vi "Create Message Accessors.vi"(6 "Enum Parameters":T1[](array[typedef]), 7 "Message parameters":T2[](array[typedef]), 8 "error in (no error)":errorcluster, 11 "Library":refnum<vi>) -> (0 "error out":errorcluster, 3 "Library":refnum<vi>)   [LabVIEW 2019, in "gRPC Template Creation Utility.lvlib"]
uses:
  gRPC Template Creation Utility.lvlib
  TypeDefs/Message Metadata (Scripting).ctl
  TypeDefs/Message Element Metadata (Scripting).ctl
  TypeDefs/Message Element Type.ctl
  TypeDefs/Enum Metadata (Scripting).ctl
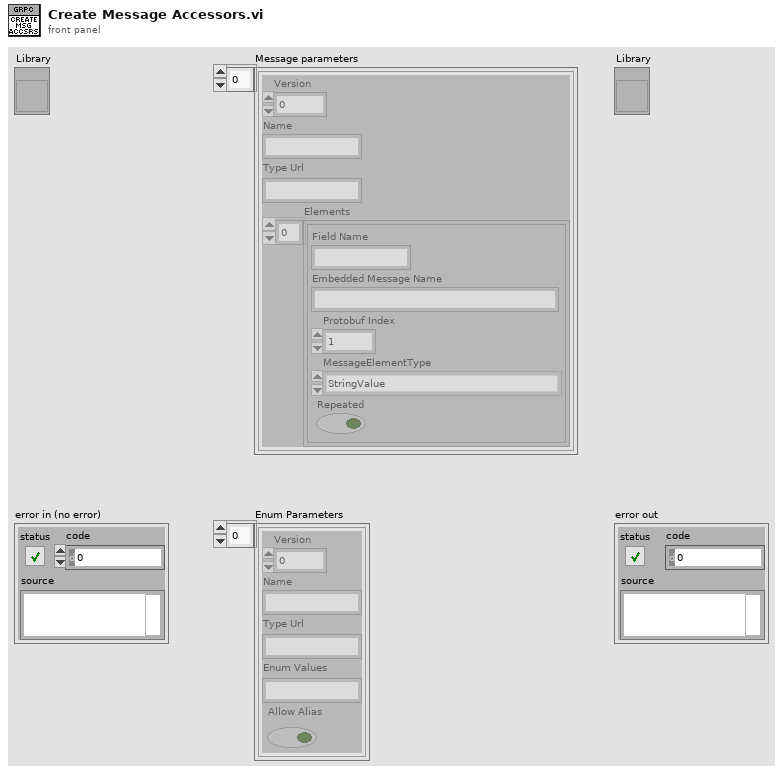
[diagram p1: front panel]
types:
  T1 = typedef "gRPC Template Creation Utility.lvlib/Enum Metadata (Scripting).ctl" = cluster{"Version":i32, "Name":string, "Type Url":string, "Enum Values":string, "Allow Alias":bool}
  T2 = typedef "gRPC Template Creation Utility.lvlib/Message Metadata (Scripting).ctl" = cluster{"Version":i32, "Name":string, "Type Url":string, "Elements":T3[]}
  T3 = typedef "gRPC Template Creation Utility.lvlib/Message Element Metadata (Scripting).ctl" = cluster{"Field Name":string, "Embedded Message Name":string, "Protobuf Index":i32, "MessageElementType":T4, "Repeated":bool}
  T4 = typedef "gRPC Template Creation Utility.lvlib/Message Element Type.ctl" = enum32{"Int32Value", "FloatValue", "DoubleValue", "BoolValue", "StringValue", "MessageValue", "Int64Value", "UInt32Value", "UInt64Value", "EnumValue", "Bytes", "Fixed64", "Fixed32", "SFixed64", "SFixed32", "SInt64", "SInt32"}
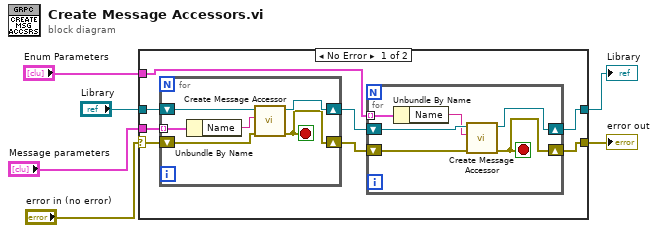
[diagram p0: block diagram]
diagram:
  n1 = case shown="No Error" "error in (no error)" {
    selector: "error in (no error)" -> [w13 w27]
    tunnel: [w7 w28] -> w6
    tunnel: "Library" -> [w12 w28]
    tunnel: [w10 w27] -> w4
    tunnel: "Message parameters" -> [w14 _]
    tunnel: "Enum Parameters" -> [w9 _]
    frame No Error {
      n2 = for {
        shift-right: [w23] -> w11
        shift-left: w13 -> [w26]
        shift-right: [w24] -> w8
        shift-left: w12 -> [w25]
        tunnel: w14 -> [w22] mode=indexing
        stop <- w23 stop-if-true
        n3 = Unbundle By Name(w22) -> ("Name"=w21:string)
        n4 = call "Create Message Accessor.vi"("error in (no error)"=w26, "Message Name"=w21, "Library"=w25) -> ("error out"=w23:errorcluster, "Library"=w24:refnum<vi>)  [unwired: 7 in]
      }
      n5 = for {
        shift-right: [w17] -> w10
        shift-left: w11 -> [w20]
        shift-right: [w18] -> w7
        shift-left: w8 -> [w19]
        tunnel: w9 -> [w16] mode=indexing
        stop <- w17 stop-if-true
        n6 = Unbundle By Name(w16) -> ("Name"=w15:string)
        n7 = call "Create Message Accessor.vi"("error in (no error)"=w20, "Message Name"=w15, "Library"=w19) -> ("error out"=w17:errorcluster, "Library"=w18:refnum<vi>)  [unwired: 7 in]
      }
    }
    frame Error {
    }
  }
  "Library" <- w6
  "error out" <- w4
